vi "Test 10  13  16  21  30  45 backwards.vi"(8 "error in (no error)":errorcluster, 11 "Test Case In":refnum<class "Day 09 Test.lvclass">) -> (0 "error out":errorcluster, 3 "Test Case Out":refnum<class "Day 09 Test.lvclass">)   [LabVIEW 2020, in "Day 09 Test.lvclass"]
uses:
  Day 09 Test.lvclass
  C:/Program Files (x86)/National Instruments/LabVIEW 2020/vi.lib/Astemes/LUnit/Test Case.lvclass
  <vilib>/Astemes/LUnit/Test Case.lvclass/Test Case.ctl
  4993e8ee-a06a-463a-9684-69129f64d5ce.vi
  <vilib>/Astemes/LUnit/Append Pass Result.vi
  <vilib>/Astemes/LUnit/Append Fail Result.vi
  <vilib>/Astemes/LUnit/Describe Comparison.vi
  <vilib>/Astemes/LUnit/Compare Variants.vi
  <vilib>/Astemes/LUnit/Variant to string.vi
  <vilib>/Utility/Data Type/Get Type Information.vi
  <vilib>/Utility/LVClass/Get LV Class Name.vi
  Measurement/Measurement.lvclass
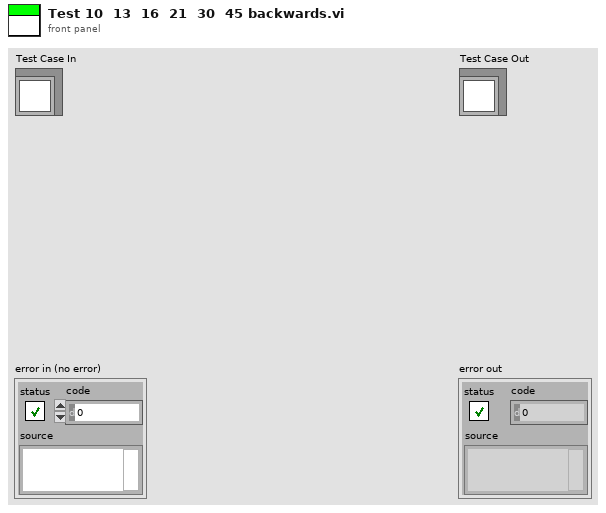
[diagram p1: front panel]
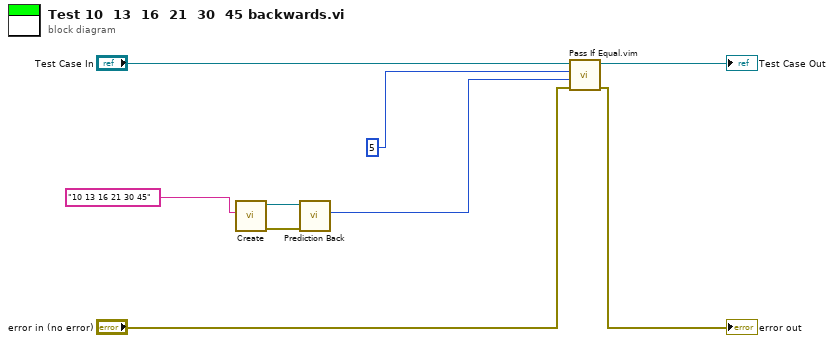
[diagram p0: block diagram]
diagram:
  n1 = call "Create.vi"("Input"="10 13 16 21 30 45") -> ("error out"=w3:errorcluster, "Measurement"=w4:refnum<class "Measurement.lvclass">)  [unwired: 9 in]
  n2 = call "Prediction Back.vi"("error in (no error)"=w3, "Measurement in"=w4) -> ("Numeric"=w2:i64)  [unwired: 7 in, 2 out]
  n3 = call "Pass If Equal.vim"("error in (no error)"="error in (no error)", "Actual"=w2, "Expected"=i64 5 ("Numeric"), "LUnit Test Case In"="Test Case In") -> ("error out"=→"error out":errorcluster, "LUnit Test Case Out"=→"Test Case Out":refnum<class "Day 09 Test.lvclass">)  [unwired: 6 in]
